vi "Color config for intensity map U16 (SubVI).vi"(8 "IntensityGraph ref in":refnum<vi>, 9 "max adjust":dbl=1.2 format="%#_13g", 10 "color":T1={"color array"=[0, 16711680, 16776960, 16448250, 16776960, 16711680, 16448250, 16448250], "num of colors"=4, "max"=150.0, "min"=100.0, "auto"=FALSE, "Zoom"=0.69999945} {"Zoom" format="%_2g"; "min" step=0.01 format="%_2f"; "max" step=0.1 format="%_3f"}, 11 "image in":u16[][](array[numeric])) -> (0 "Zoom":sgl, 1 "max value":u16=2057, 3 "image out":u16[][](array[numeric]))   [LabVIEW 2024]
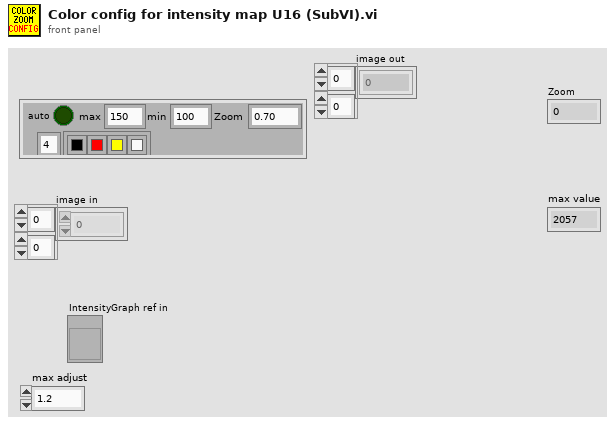
[diagram p1: front panel]
types:
  T1 = cluster{"color array":u32[], "num of colors":i32, "max":dbl, "min":dbl, "auto":bool, "Zoom":sgl}
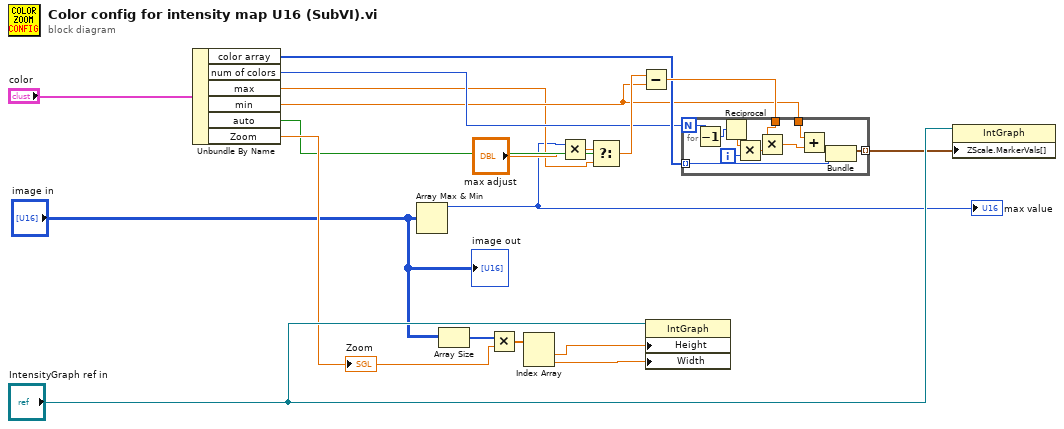
[diagram p0: block diagram]
diagram:
  n1 = Unbundle By Name("color") -> ("color array"=w7:u32[], "num of colors"=w6:i32, "max"=w3:dbl, "min"=w5:dbl, "auto"=w17:bool, "Zoom"=w18:sgl)
  "Zoom" <- w18
  n2 = Array Max & Min(array="image in") -> (max value=w2:u16)  [unwired: 3 out]
  "max value" <- w2
  n3 = Array Size(array="image in") -> (size(s)=w14:i32[])
  n4 = Multiply(x=w14, y=w18) -> (x*y=w12:sgl[])
  n5 = Index Array(array=w12) -> (element #1=w13:sgl, element #2=w15:sgl)  [unwired: 2 in]
  n6 = Multiply(x=w2, y="max adjust") -> (x*y=w1:dbl)
  n7 = Select(t=w1, s=w17, f=w3) -> (s? t:f=w9:dbl)
  n8 = Subtract(x=w9, y=w5) -> (x-y=w8:dbl)
  n9 = property on="Property Node" class="IntGraph"(reference="IntensityGraph ref in", "Height"=w13, "Width"=w15) -> ()  [unwired: 1 in, 2 out]
  n10 = for {
    N: w6 -> [w24]
    tunnel: w8 -> [w28]
    tunnel: [w26] -> w11 mode=indexing
    tunnel: w7 -> [w25] mode=indexing
    tunnel: w5 -> [w20]
    i -> [w30]
    n11 = Decrement(x=w24) -> (x-1=w23:i32)
    n12 = Reciprocal(x=w23) -> (1/x=w22:dbl)
    n13 = Multiply(x=w22, y=w30) -> (x*y=w29:dbl)
    n14 = Multiply(x=w28, y=w29) -> (x*y=w27:dbl)
    n15 = Add(x=w20, y=w27) -> (x+y=w21:dbl)
    n16 = Bundle(w21, w25) -> (w26:cluster{dbl, u32})  [unwired: 1 in]
  }
  n17 = property on="Property Node" class="IntGraph"(reference="IntensityGraph ref in", "ZScale.MarkerVals[]"=w11) -> ()  [unwired: 1 in, 2 out]
  "image out" <- "image in"
